vi "PrintDebugInfo.vi"(8 "error in (no error)":errorcluster, 11 "CLabVIEWItem in":refnum<class "CLabVIEWItem.lvclass">) -> (0 "error out":errorcluster, 1 "Debug string":string, 3 "CLabVIEWItem out":refnum<class "CLabVIEWItem.lvclass">)   [LabVIEW 2020, in "LabVIEWItem.lvlib" / "CLabVIEWItem.lvclass"]
uses:
  CLabVIEWItem.lvclass
  CLabVIEWItem.lvclass/CLabVIEWItem.ctl
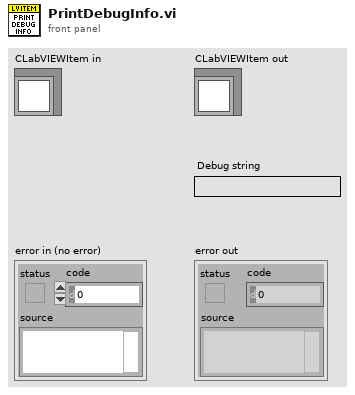
[diagram p1: front panel]
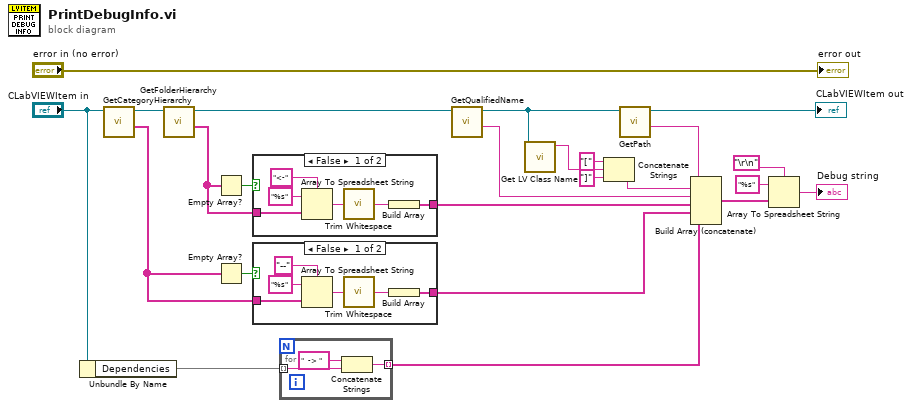
[diagram p0: block diagram]
diagram:
  n1 = Unbundle By Name("CLabVIEWItem in") -> ("Dependencies"=w24:set{string})
  n2 = call-dynamic "GetCategoryHierarchy.vi"("CLabVIEWItem in"="CLabVIEWItem in") -> ("Category hierarchy[]"=w8:string[], "CLabVIEWItem out"=w13:refnum<class "CLabVIEWItem.lvclass">)  [unwired: 8 in, 1 out]
  n3 = call-dynamic "GetFolderHierarchy.vi"("CLabVIEWItem in"=w13) -> ("Folder hierarchy[]"=w11:string[], "CLabVIEWItem out"=w15:refnum<class "CLabVIEWItem.lvclass">)  [unwired: 8 in, 1 out]
  n4 = Empty Array?(array=w11) -> (empty?=w10:bool)
  n5 = Empty Array?(array=w8) -> (empty?=w9:bool)
  n6 = case shown="False" w10 {
    tunnel: w11 -> [w29 _]
    tunnel: [w25 _] -> w12
    frame False {
      n7 = Array To Spreadsheet String(delimiter (Tab)="<-", array=w29, 3:"%s" ("format string")) -> (spreadsheet string=w27:string)
      n8 = call <vilib>:"Trim Whitespace.vi"("string"=w27) -> ("trimmed string"=w26:string)  [unwired: 1 in]
      n9 = Build Array(w26) -> (w25:string[])
    }
    frame True {
    }
  }
  n10 = case shown="False" w9 {
    tunnel: w8 -> [w35 _]
    tunnel: [w31 _] -> w7
    frame False {
      n11 = Array To Spreadsheet String(delimiter (Tab)="--", array=w35, 3:"%s" ("format string")) -> (spreadsheet string=w33:string)
      n12 = call <vilib>:"Trim Whitespace.vi"("string"=w33) -> ("trimmed string"=w32:string)  [unwired: 1 in]
      n13 = Build Array(w32) -> (w31:string[])
    }
    frame True {
    }
  }
  n14 = for {
    tunnel: w24 -> [w39] mode=indexing
    tunnel: [w38] -> w22 mode=indexing
    n15 = Concatenate Strings("  -> " ("string"), w39) -> (w38:string)
  }
  n16 = call-dynamic "GetQualifiedName.vi"("CLabVIEWItem in"=w15) -> ("Qualified name"=w17:string, "CLabVIEWItem out"=w6:refnum<class "CLabVIEWItem.lvclass">)  [unwired: 8 in, 1 out]
  n17 = call <vilib>:"Get LV Class Name.vi"("object"=w6) -> ("class name"=w5:string)  [unwired: 9 in, 1 out]
  n18 = Concatenate Strings("[" ("string"), w5, "]" ("string")) -> (w4:string)
  n19 = call-dynamic "GetPath.vi"("CLabVIEWItem in"=w6) -> ("Path"=w1:string, "CLabVIEWItem out"=→"CLabVIEWItem out":refnum<class "CLabVIEWItem.lvclass">)  [unwired: 8 in, 1 out]
  n20 = Build Array (concatenate)(w1, w4, w17, w12, w7, w22) -> (w18:string[])
  n21 = Array To Spreadsheet String(delimiter (Tab)="\r\n", array=w18, 3:"%s" ("format string")) -> (spreadsheet string=→"Debug string":string)
  "error out" <- "error in (no error)"
